vi "Eval Parsed Formula Node.vi"(2 "error in (no error)":errorcluster, 3 "Parsed Formula Node":T1 {"Y Values" format="%.2f"}, 4 "Input Values":dbl[](array[numeric]) format="%.2f") -> (0 "error out":errorcluster, 1 "Output Values":dbl[](array[numeric]) format="%.2f")   [LabVIEW 2017, in "NI_Gmath.lvlib"]
doc: "Separates the parsing process from the evaluating process of the Eval Formula Node VI and improves the run-time behavior of a program containing Eval Formula Node VIs at different locations."
uses:
  NI_Gmath.lvlib
panel:
  # "Example:\n\n See Parse Formula Node.vi!"
  # "operator"
  # "register1"
  # "register2"
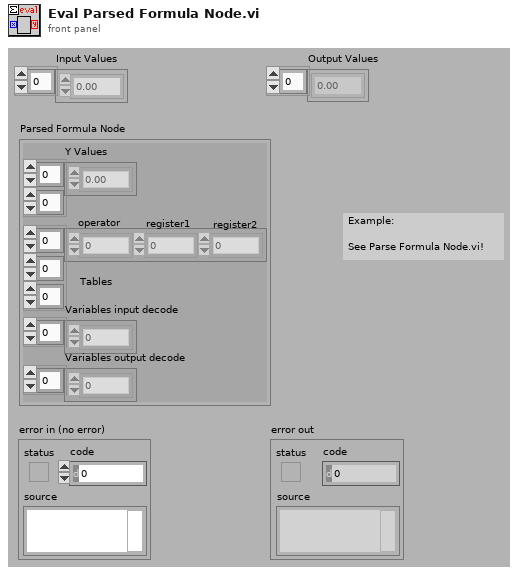
[diagram p1: front panel]
types:
  T1 = cluster{"Y Values":dbl[][], "Tables":i32[][][], "Variables input decode":i32[], "Variables output decode":i32[]}
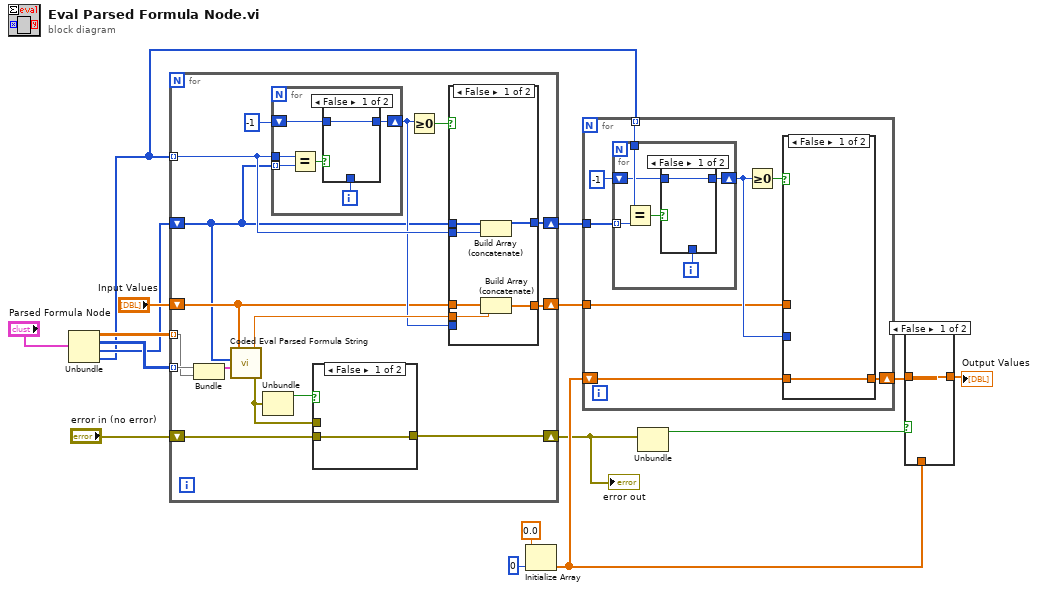
[diagram p0: block diagram]
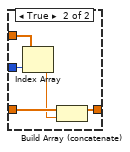
[diagram p4: hidden frame]
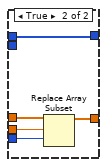
[diagram p6: hidden frame]
diagram:
  n1 = Unbundle("Parsed Formula Node") -> ("Y Values"=w9:dbl[][], "Tables"=w8:i32[][][], "Variables input decode"=w7:i32[], "Variables output decode"=w6:i32[])
  n2 = for {
    shift-right: [w30] -> w13
    shift-left: w7 -> [w20]
    shift-right: [w28] -> w12
    shift-left: "Input Values" -> [w21]
    tunnel: w8 -> [w18] mode=indexing
    tunnel: w9 -> [w17] mode=indexing
    tunnel: w6 -> [w29] mode=indexing
    shift-right: [w23] -> w1
    shift-left: "error in (no error)" -> [w22]
    n3 = Bundle("Tables"=w18, "Y Values"=w17) -> (w19:cluster{"Tables":i32[][], "Y Values":dbl[]})  [unwired: 1 in]
    n4 = call "Coded Eval Parsed Formula String.vi"("Parsed Formula"=w19, "Variables"=w20, "X Values"=w21) -> ("error out"=w24:errorcluster, "y value"=w27:dbl)  [unwired: 1 in]
    n5 = Unbundle(w24) -> ("status"=w25:bool)  [unwired: 2 out]
    n6 = for {
      shift-right: [w47] -> w26
      shift-left: -1 -> [w48]
      tunnel: w29 -> [w51]
      tunnel: w20 -> [w50] mode=indexing
      i -> [w46]
      n7 = Equal?(x=w51, y=w50) -> (x = y?=w49:bool)
      n8 = case shown="False" w49 {
        tunnel: w48 -> [w52 _]
        tunnel: [w52 w53] -> w47
        tunnel: w46 -> [_ w53]
        frame False {
        }
        frame True {
        }
      }
    }
    n9 = case shown="False" w25 {
      tunnel: w24 -> [_ w34]
      tunnel: [w33 w34] -> w23
      tunnel: w22 -> [w33 _]
      frame False {
      }
      frame True {
      }
    }
    n10 = Greater Or Equal To 0?(x=w26) -> (x >= 0?=w31:bool)
    n11 = case shown="False" w31 {
      tunnel: w20 -> [w40 w45]
      tunnel: [w39 w45] -> w30
      tunnel: w29 -> [w38 _]
      tunnel: w21 -> [w37 w44]
      tunnel: [w36 w43] -> w28
      tunnel: w27 -> [w35 w42]
      tunnel: w26 -> [_ w41]
      frame False {
        n12 = Build Array (concatenate)(w40, w38) -> (w39:i32[])
        n13 = Build Array (concatenate)(w37, w35) -> (w36:dbl[])
      }
      frame True {
        n14 = Replace Array Subset(array=w44, new element=w42, index=w41) -> (w43:dbl[])
      }
    }
  }
  "error out" <- w1
  n15 = Initialize Array(0.0, 0) -> (w4:dbl[])
  n16 = for {
    shift-right: [w57] -> w10
    shift-left: w4 -> [w56]
    tunnel: w13 -> [w61]
    tunnel: w6 -> [w60] mode=indexing
    tunnel: w12 -> [w54]
    n17 = for {
      tunnel: w61 -> [w67] mode=indexing
      tunnel: w60 -> [w66]
      shift-right: [w64] -> w55
      shift-left: -1 -> [w65]
      i -> [w63]
      n18 = Equal?(x=w66, y=w67) -> (x = y?=w62:bool)
      n19 = case shown="False" w62 {
        tunnel: w65 -> [w68 _]
        tunnel: [w68 w69] -> w64
        tunnel: w63 -> [_ w69]
        frame False {
        }
        frame True {
        }
      }
    }
    n20 = Greater Or Equal To 0?(x=w55) -> (x >= 0?=w58:bool)
    n21 = case shown="False" w58 {
      tunnel: [w70 w75] -> w57
      tunnel: w56 -> [w70 w74]
      tunnel: w55 -> [_ w73]
      tunnel: w54 -> [_ w72]
      frame False {
      }
      frame True {
        n22 = Index Array(array=w72, index=w73) -> (element=w71:dbl)
        n23 = Build Array (concatenate)(w74, w71) -> (w75:dbl[])
      }
    }
  }
  n24 = Unbundle(w1) -> ("status"=w11:bool)  [unwired: 2 out]
  n25 = case shown="False" w11 {
    tunnel: w10 -> [w76 _]
    tunnel: [w76 w77] -> w5
    tunnel: w4 -> [_ w77]
    frame False {
    }
    frame True {
    }
  }
  "Output Values" <- w5
